vi "generate_DAC_voltages_withSubVis.vi"(7 "focus mode?":bool, 8 "derived values":T1, 9 "scan specification":T4={"x amplitude"=0, "x resolution (pixels)"=0, "x offset fly-forward (iterations)"=0, "x offset fly-back (iterations)"=0, "y resolution (nr. of lines)"=0, "y step size"=0, "iterations per pixel"=0, "number of frames"=0, "y offset (pixels)"=0, "number of y-brake lines  (before y-fly-back)"=0, "number y-brake lines (after y-fly-back)"=0, "number of y-fly-back steps"=8, "lines per z step"=0, "number of z/intensity tuples"=0, "number of repetitions (volumes or planes)"=0, "z step size derived"=0, "choose the beginning of z scan"=FALSE, "number of frames (settings)"=0, "FPGA trajectory?"=FALSE}, 10 "counter cluster in":T2, 11 "resonant trigger":bool) -> (0 "acquire?":bool, 1 "fly-back acquisition phase?":bool, 2 "counter cluster out":T2, 3 "DAC voltages":T3 {"ch6" max=4095 step=1; "ch5" max=4095 step=1; "ch4" max=4095 step=1; "ch3" max=4095 step=1; "ch2" max=4095 step=1; "ch1" max=4095 step=1; "ch0" max=4095 step=1})   [LabVIEW 2010]
uses:
  scan_specification_cluster.ctl
  common_typedefs/DAC_voltage_cluster.ctl
  counter_cluster.ctl
  derived_values_cluster.ctl
panel:
  out "coerced(x) 2":u16
  out "unsigned 16bit integer":u16
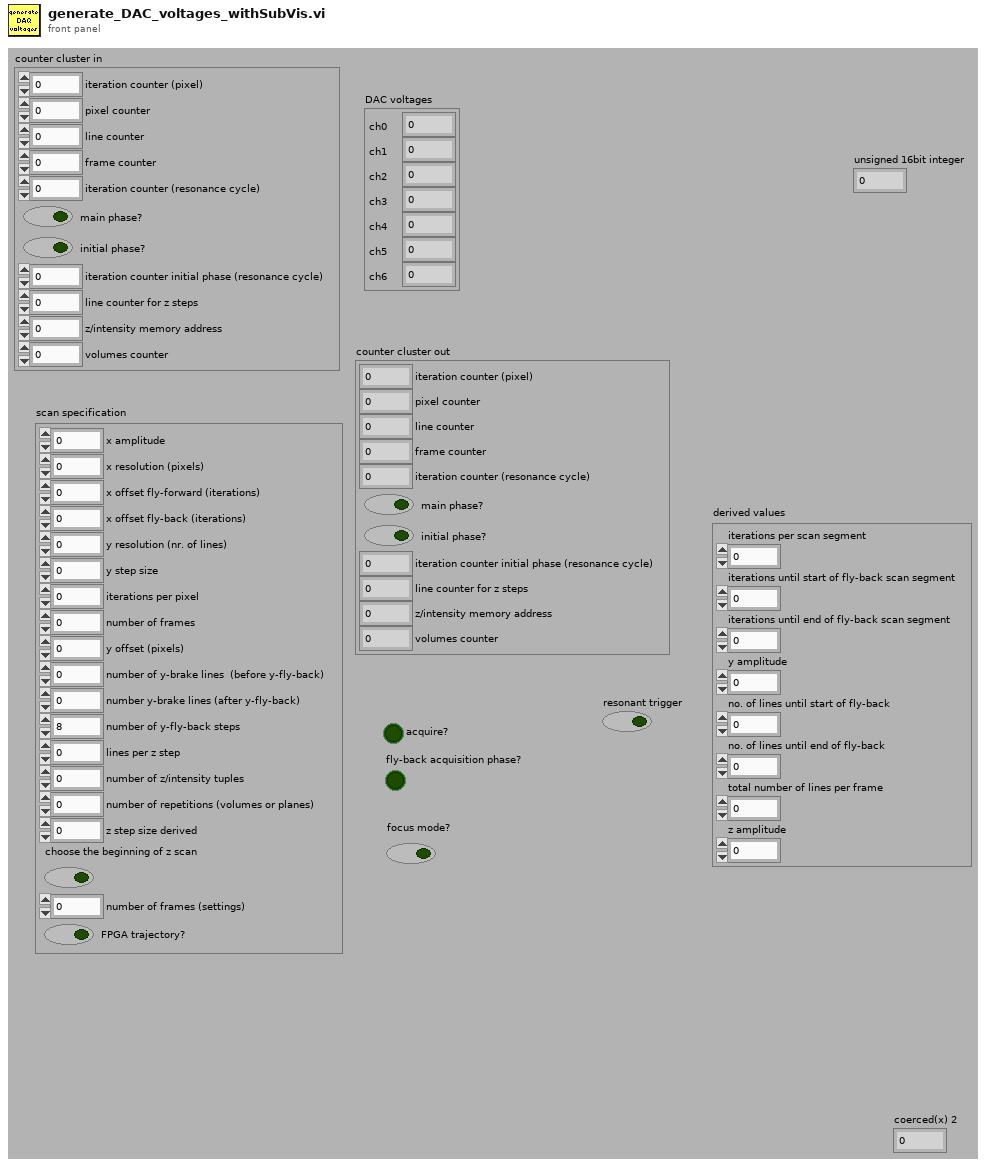
[diagram p1: front panel]
types:
  T1 = typedef "derived_values_cluster.ctl" = cluster{"iterations per scan segment":u16, "iterations until start of fly-back scan segment":u16, "iterations until end of fly-back scan segment":u16, "y amplitude":u16, "no. of lines until start of fly-back":u16, "no. of lines until end of fly-back":u16, "total number of lines per frame ":u16, "z amplitude":u16}
  T2 = typedef "counter_cluster.ctl" = cluster{"iteration counter (pixel)":u16, "pixel counter":u16, "line counter":u16, "frame counter":u16, "iteration counter (resonance cycle)":u16, "main phase?":bool, "initial phase?":bool, "iteration counter initial phase (resonance cycle)":u16, "line counter for z steps":u16, "z/intensity memory address":u32, "volumes counter":u16}
  T3 = typedef "DAC_voltage_cluster.ctl" = cluster{"ch0":u16, "ch1":i16, "ch2":i16, "ch3":u16, "ch4":u16, "ch5":u16, "ch6":u16}
  T4 = typedef "scan_specification_cluster.ctl" = cluster{"x amplitude":u16, "x resolution (pixels)":u16, "x offset fly-forward (iterations)":u16, "x offset fly-back (iterations)":u16, "y resolution (nr. of lines)":u16, "y step size":u16, "iterations per pixel":u16, "number of frames":i32, "y offset (pixels)":u16, "number of y-brake lines  (before y-fly-back)":u16, "number y-brake lines (after y-fly-back)":u16, "number of y-fly-back steps":u16, "lines per z step":u16, "number of z/intensity tuples":u16, "number of repetitions (volumes or planes)":i32, "z step size derived":u16, "choose the beginning of z scan":bool, "number of frames (settings)":i32, "FPGA trajectory?":bool}
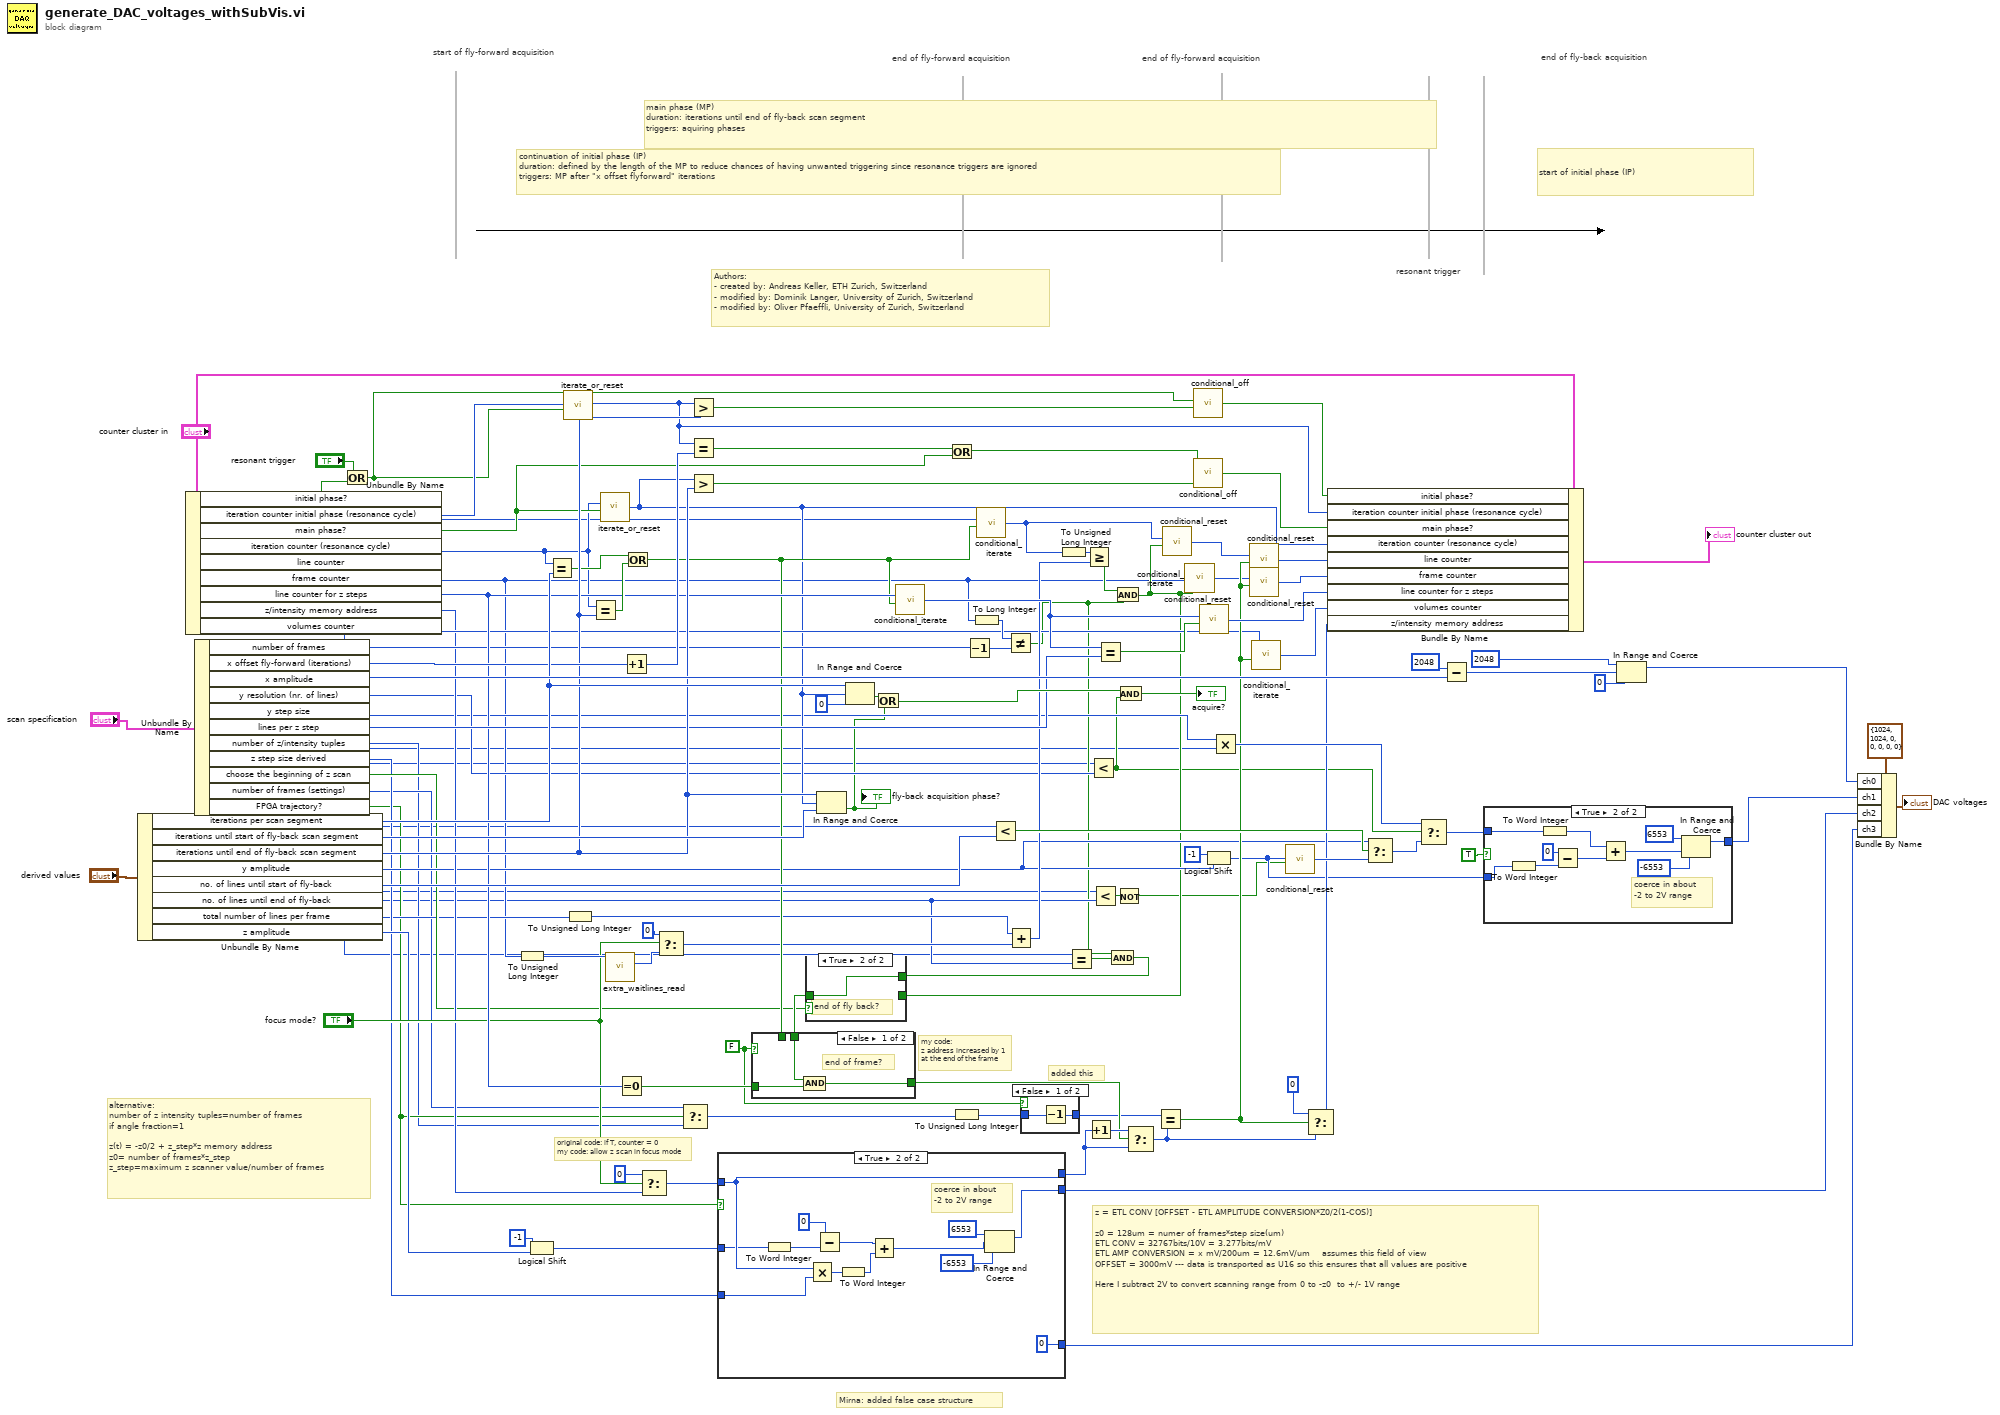
[diagram p0: block diagram]
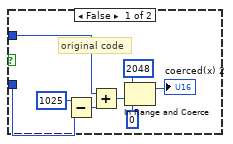
[diagram p3: hidden frame]
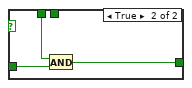
[diagram p5: hidden frame]
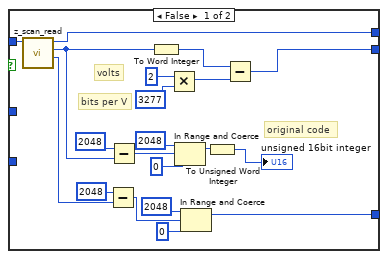
[diagram p6: hidden frame]
diagram:
  w3 = FALSE
  # "added this"
  # "z = ETL CONV [OFFSET - ETL AMPLITUDE CONVERSION*Z0/2(1-COS)]\n\nz0 = 128um = numer of frames*step size(um)\nETL CONV = 32767bits/10V = 3.277bits/mV\nETL AMP CONVERSION = x mV/200um = 12.6mV/um    assumes this field of view\nOFFSET = 3000mV --- data is transported as U16 so this ensures that all values are positive\n\nHere I subtract 2V to convert scanning range from 0 to -z0  to +/- 1V range"
  # "my code:\nz address increased by 1\nat the end of the frame"
  # "alternative:\nnumber of z intensity tuples=number of frames\nif angle fraction=1\n\nz(t) = -z0/2 + z_step*z memory address\nz0= number of frames*z_step\nz_step=maximum z scanner value/number of frames"
  # "original code: if T, counter = 0\nmy code: allow z scan in focus mode"
  # "Mirna: added false case structure"
  # "start of initial phase (IP)"
  # "continuation of initial phase (IP)\nduration: defined by the length of the MP to reduce chances of having unwanted triggering since resonance triggers are ignored\ntriggers: MP after \"x offset flyforward\" iterations"
  # "end of fly-back acquisition"
  # "end of fly-forward acquisition"
  # "end of fly-forward acquisition"
  # "start of fly-forward acquisition"
  # "main phase (MP)\nduration: iterations until end of fly-back scan segment\ntriggers: aquiring phases"
  # "resonant trigger"
  # "Authors: \n- created by: Andreas Keller, ETH Zurich, Switzerland\n- modified by: Dominik Langer, University of Zurich, Switzerland\n- modified by: Oliver Pfaeffli, University of Zurich, Switzerland"
  n1 = Unbundle By Name("derived values") -> ("iterations per scan segment"=w91:u16, "iterations until start of fly-back scan segment"=w94:u16, "iterations until end of fly-back scan segment"=w78:u16, "y amplitude"=w33:u16, "no. of lines until start of fly-back"=w82:u16, "no. of lines until end of fly-back"=w8:u16, "total number of lines per frame"=w26:u16, "z amplitude"=w31:u16)
  n2 = Unbundle By Name("counter cluster in") -> ("initial phase?"=w93:bool, "iteration counter initial phase (resonance cycle)"=w89:u16, "main phase?"=w45:bool, "iteration counter (resonance cycle)"=w36:u16, "line counter"=w2:u16, "frame counter"=w25:u16, "line counter for z steps"=w71:u16, "z/intensity memory address"=w39:u32, "volumes counter"=w50:u16)
  n3 = Unbundle By Name("scan specification") -> ("number of frames"=w57:i32, "x offset fly-forward (iterations)"=w81:u16, "x amplitude"=w98:u16, "y resolution (nr. of lines)"=w37:u16, "y step size"=w32:u16, "lines per z step"=w75:u16, "number of z/intensity tuples"=w10:u16, "z step size derived"=w27:u16, "choose the beginning of z scan"=w28:bool, "number of frames (settings)"=w11:i32, "FPGA trajectory?"=w12:bool)
  n4 = Or(x="resonant trigger", y=w93) -> (x .or. y?=w87:bool)
  n5 = To Unsigned Long Integer(number=w25) -> (unsigned 32bit integer=w63:u32)
  n6 = Logical Shift(y=i16 -1 ("n"), x=w31) -> (x << y=w47:u16)
  n7 = Equal?(x=w36, y=w91) -> (x = y?=w76:bool)
  n8 = call "iterate_or_reset.vi"("iterate?"=w87, "number in"=w89) -> ("number out"=w22:u16)  [unwired: 4 in]
  n9 = To Unsigned Long Integer(number=w26) -> (unsigned 32bit integer=w23:u32)
  n10 = Equal?(x=w36, y=w78) -> (x = y?=w77:bool)
  n11 = call "iterate_or_reset.vi"("iterate?"=w45, "number in"=w36) -> ("number out"=w44:u16)  [unwired: 4 in]
  n12 = call "extra_waitlines_read.vi"("address extra waitlines IN"=w63) -> ("extra waitline data"=w5:u32)  [unwired: 9 in, 1 out]
  n13 = Equal To 0?(x=w71) -> (x = 0?=w66:bool)
  n14 = Increment(x=w81) -> (x+1=w80:u16)
  n15 = Or(x=w76, y=w77) -> (x .or. y?=w65:bool)
  n16 = Select(t=u32 0, s="focus mode?", f=w39) -> (s? t:f=w40:u32)
  n17 = Select(t=u32 0, s="focus mode?", f=w5) -> (s? t:f=w52:u32)
  n18 = Select(t=w11, s=w12, f=w10) -> (s? t:f=w38:i32)
  n19 = Greater?(x=w22, y=w78) -> (0:w79:bool)
  n20 = Equal?(x=w22, y=w80) -> (x = y?=w88:bool)
  n21 = Greater?(x=w44, y=w78) -> (0:w85:bool)
  n22 = case shown="True" w12 {
    tunnel: [w126 u16 0 ("intensity")] -> w42
    tunnel: [w133 w143] -> w64
    tunnel: [w117 w134] -> w41
    tunnel: w40 -> [w132 w143]
    tunnel: w47 -> [_ w135]
    tunnel: w27 -> [_ w144]
    frame False {
      # "bits per V"
      # "volts"
      # "original code"
      n23 = call "z_scan_read.vi"("address in"=w132) -> ("intensity"=w129:u16, "z-value"=w119:i16, "address out"=w133:u32)  [unwired: 8 in]
      n24 = Subtract(x=i16 2048, y=w129) -> (x-y=w125:u16)
      n25 = Subtract(x=i16 2048, y=w119) -> (x-y=w121:i16)
      n26 = To Word Integer(number=w119) -> (16bit integer=w118:i16)
      n27 = Multiply(x=i16 2 ("y"), y=i16 3277) -> (x*y=w115:i16)
      n28 = In Range and Coerce(upper limit=i16 2048, x=w121, lower limit=i16 0) -> (coerced(x)=w122:i16)  [unwired: 1 out]
      n29 = In Range and Coerce(upper limit=u16 2048, x=w125, lower limit=u16 0) -> (coerced(x)=w126:u16)  [unwired: 1 out]
      n30 = To Unsigned Word Integer(number=w122) -> (unsigned 16bit integer=→"unsigned 16bit integer":u16)
      n31 = Subtract(x=w118, y=w115) -> (x-y=w117:i16)
    }
    frame True {
      # "coerce in about\n-2 to 2V range"
      n32 = To Word Integer(number=w135) -> (16bit integer=w140:i16)
      n33 = Multiply(x=w143, y=w144) -> (x*y=w141:u32)
      n34 = Subtract(x=i16 0, y=w140) -> (x-y=w142:i16)
      n35 = To Word Integer(number=w141) -> (16bit integer=w139:i16)
      n36 = Add(x=w142, y=w139) -> (x+y=w136:i16)
      n37 = In Range and Coerce(upper limit=i16 6553, x=w136, lower limit=i16 -6553) -> (coerced(x)=w134:i16)  [unwired: 1 out]
    }
  }
  n38 = In Range and Coerce(upper limit=w78, x=w44, lower limit=w94) -> (In Range?=w15:bool)  [unwired: 1 out]
  "fly-back acquisition phase?" <- w15
  n39 = In Range and Coerce(upper limit=w91, x=w44, lower limit=u16 0) -> (In Range?=w106:bool)  [unwired: 1 out]
  n40 = Or(x=w106, y=w15) -> (x .or. y?=w97:bool)
  n41 = call "conditional_iterate.vi"("iterate?"=w65, "number in"=w71) -> ("number out"=w72:u16)  [unwired: 4 in]
  n42 = Or(x=w88, y=w45) -> (x .or. y?=w46:bool)
  n43 = To Unsigned Long Integer(number=w38) -> (unsigned 32bit integer=w69:u32)
  n44 = Decrement(x=w57) -> (x-1=w56:i32)
  n45 = To Long Integer(number=w25) -> (32bit integer=w55:i32)
  n46 = call "conditional_iterate.vi"("iterate?"=w65, "number in"=w2) -> ("number out"=w7:u16)  [unwired: 4 in]
  n47 = Less?(x=w2, y=w82) -> (x < y?=w112:bool)
  n48 = Not Equal?(x=w55, y=w56) -> (x != y?=w6:bool)
  n49 = Add(x=w23, y=w52) -> (x+y=w53:u32)
  n50 = case shown="False" w3 {
    tunnel: w69 -> [w148 w149]
    tunnel: [w147 w149] -> w4
    frame False {
      n51 = Decrement(x=w148) -> (x-1=w147:u32)
    }
    frame True {
    }
  }
  n52 = To Unsigned Long Integer(number=w7) -> (unsigned 32bit integer=w9:u32)
  n53 = Equal?(x=w2, y=w8) -> (x = y?=w13:bool)
  n54 = Greater Or Equal?(x=w9, y=w53) -> (x >= y?=w58:bool)
  n55 = Increment(x=w64) -> (x+1=w70:u32)
  n56 = Less?(x=w2, y=w37) -> (x < y?=w18:bool)
  n57 = Less?(x=w2, y=w8) -> (x < y?=w96:bool)
  n58 = Equal?(x=w72, y=w75) -> (x = y?=w73:bool)
  n59 = And(x=w6, y=w13) -> (x .and. y?=w14:bool)
  n60 = And(x=w58, y=w6) -> (x .and. y?=w30:bool)
  n61 = case shown="True" w28 {
    tunnel: w14 -> [_ w151]
    tunnel: w30 -> [w150 _]
    tunnel: [w150 w151] -> w29
    frame False {
      # "end of frame?"
    }
    frame True {
      # "end of fly back?"
    }
  }
  n62 = case shown="False" w3 {
    tunnel: w66 -> [w154 w157]
    tunnel: w65 -> [_ w156]
    tunnel: [w153 w155] -> w24
    tunnel: w29 -> [w152 _]
    frame False {
      # "end of frame?"
      n63 = And(x=w152, y=w154) -> (x .and. y?=w153:bool)
    }
    frame True {
      n64 = And(x=w156, y=w157) -> (x .and. y?=w155:bool)
    }
  }
  n65 = Not(x=w96) -> (.not. x?=w16:bool)
  n66 = And(x=w97, y=w18) -> (x .and. y?=→"acquire?":bool)
  n67 = Select(t=w70, s=w24, f=w64) -> (s? t:f=w68:u32)
  n68 = Equal?(x=w4, y=w68) -> (x = y?=w54:bool)
  n69 = call "conditional_reset.vi"("reset?"=w30, "number in"=w7) -> ("number out"=w60:u16)  [unwired: 4 in]
  n70 = call "conditional_iterate.vi"("iterate?"=w30, "number in"=w25) -> ("number out"=w34:u16)  [unwired: 4 in]
  n71 = call "conditional_off.vi"("switch off?"=w79, "boolean in"=w87) -> ("boolean out"=w86:bool)  [unwired: 4 in]
  n72 = call "conditional_off.vi"("switch off?"=w85, "boolean in"=w46) -> ("boolean out"=w84:bool)  [unwired: 4 in]
  n73 = call "conditional_reset.vi"("reset?"=w73, "number in"=w72) -> ("number out"=w74:u16)  [unwired: 4 in]
  n74 = Logical Shift(y=i16 -1 ("n"), x=w33) -> (x << y=w17:u16)
  n75 = Multiply(x=w32, y=w2) -> (x*y=w111:u16)
  n76 = call "conditional_reset.vi"("reset?"=w54, "number in"=w60) -> ("number out"=w59:u16)  [unwired: 4 in]
  n77 = call "conditional_reset.vi"("reset?"=w54, "number in"=w34) -> ("number out"=w35:u16)  [unwired: 4 in]
  n78 = call "conditional_iterate.vi"("iterate?"=w54, "number in"=w50) -> ("number out"=w61:u16)  [unwired: 4 in]
  n79 = call "conditional_reset.vi"("reset?"=w16, "number in"=w17) -> ("number out"=w83:u16)  [unwired: 4 in]
  n80 = Select(t=u32 0, s=w54, f=w68) -> (s? t:f=w62:u32)
  n81 = Bundle By Name(cluster="counter cluster in", "initial phase?"=w86, "iteration counter initial phase (resonance cycle)"=w22, "main phase?"=w84, "iteration counter (resonance cycle)"=w44, "line counter"=w59, "frame counter"=w35, "line counter for z steps"=w74, "volumes counter"=w61, "z/intensity memory address"=w62) -> (→"counter cluster out":T2)
  n82 = Select(t=w33, s=w112, f=w83) -> (s? t:f=w19:u16)
  n83 = Select(t=w111, s=w18, f=w19) -> (s? t:f=w21:u16)
  n84 = Subtract(x=u16 2048, y=w98) -> (x-y=w102:u16)
  n85 = case shown="True" TRUE {
    tunnel: [_ w168] -> w43
    tunnel: w17 -> [w158 w167]
    tunnel: w21 -> [w159 w166]
    frame False {
      # "original code"
      n86 = Subtract(x=u16 1025, y=w158) -> (x-y=w161:u16)
      n87 = Add(x=w159, y=w161) -> (x+y=w160:u16)
      n88 = In Range and Coerce(upper limit=u16 2048, x=w160, lower limit=u16 0) -> (coerced(x)=→"coerced(x) 2":u16)  [unwired: 1 out]
    }
    frame True {
      # "coerce in about\n-2 to 2V range"
      n89 = To Word Integer(number=w167) -> (16bit integer=w173:i16)
      n90 = To Word Integer(number=w166) -> (16bit integer=w172:i16)
      n91 = Subtract(x=i16 0, y=w173) -> (x-y=w174:i16)
      n92 = Add(x=w172, y=w174) -> (x+y=w169:i16)
      n93 = In Range and Coerce(upper limit=i16 6553, x=w169, lower limit=i16 -6553) -> (coerced(x)=w168:i16)  [unwired: 1 out]
    }
  }
  n94 = In Range and Coerce(upper limit=u16 2048, x=w102, lower limit=u16 0) -> (coerced(x)=w101:u16)  [unwired: 1 out]
  n95 = Bundle By Name(cluster=T3 {"ch0"=1024, "ch1"=1024, "ch2"=0, "ch3"=0, "ch4"=0, "ch5"=0, "ch6"=0} ("DAC voltage"), "ch0"=w101, "ch1"=w43, "ch2"=w41, "ch3"=w42) -> (→"DAC voltages":T3)
